vi "DestroyProtectedEvents.vi"(8 "error in (no error)":errorcluster, 11 "SMO":refnum<class "SMO.lvclass">) -> (0 "error out":errorcluster, 3 "SMO out":refnum<class "SMO.lvclass">)   [LabVIEW 2019, in "SMO.lvclass"]
doc: "JKI State Machine Objects (SMO) 1.3.0.56\nJKI - JKI\nCopyright (c) 2017, JKI"
uses:
  SMO.lvclass
panel:
  # "For instructions on how to use the JKI State Machine Objects, examples and video tutorials, visit:\nhttp://jki.net/state-machine-objects/\n\nJKI State Machine Objects™\nhttp://jki.net/state-machine-objects/\nCopyright (C) 2005-2015, JKI <info@jki.net>\nALL RIGHTS RESERVED"
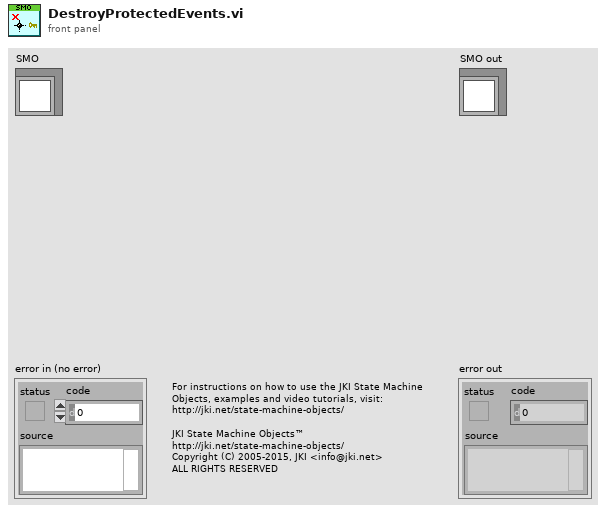
[diagram p1: front panel]
types:
  T1 = typedef "SMO.lvclass/Protected Events.ctl" = cluster{"StopProcesses":refnum<user-event>, "AbortProcesses":refnum<user-event>, "Config Changed":refnum<user-event>, "Dependency":refnum<user-event>}
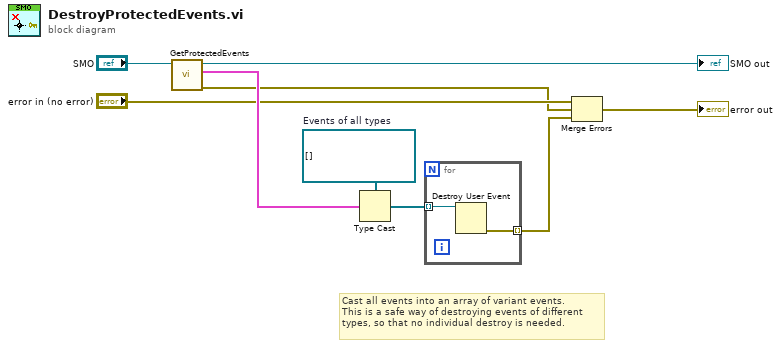
[diagram p0: block diagram]
diagram:
  w6 = refnum<user-event>[] []  # Events of all types
  # "Cast all events into an array of variant events.\nThis is a safe way of destroying events of different\ntypes, so that no individual destroy is needed."
  n1 = call "GetProtectedEvents.vi"("SMO"="SMO") -> ("error out"=w1:errorcluster, "SMO Protected Events"=w5:T1, "SMO out"=→"SMO out":refnum<class "SMO.lvclass">)  [unwired: 8 in]
  n2 = Type Cast(type=w6, x=w5) -> (*(type *) &x=w7:refnum<user-event>[])
  n3 = for {
    tunnel: w7 -> [w11] mode=indexing
    tunnel: [w10] -> w2 mode=indexing
    n4 = Destroy User Event(user event=w11) -> (error out=w10:errorcluster)  [unwired: 1 in]
  }
  n5 = Merge Errors("error in (no error)", w1, w2) -> (→"error out":errorcluster)
